vi "Readtext.vi"(8 "error in (no error)":errorcluster, 11 "object in":refnum<class "stream Message.lvclass">) -> (0 "error out":errorcluster, 2 "text":string, 3 "object out":refnum<class "stream Message.lvclass">)   [LabVIEW 2018, in "ClientMessaging.lvlib" / "stream Message.lvclass"]
uses:
  stream Message.lvclass
  stream Message.lvclass/stream Message.ctl
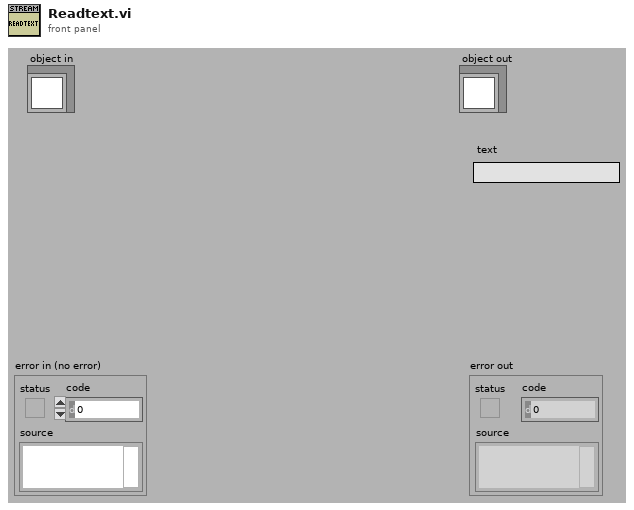
[diagram p1: front panel]
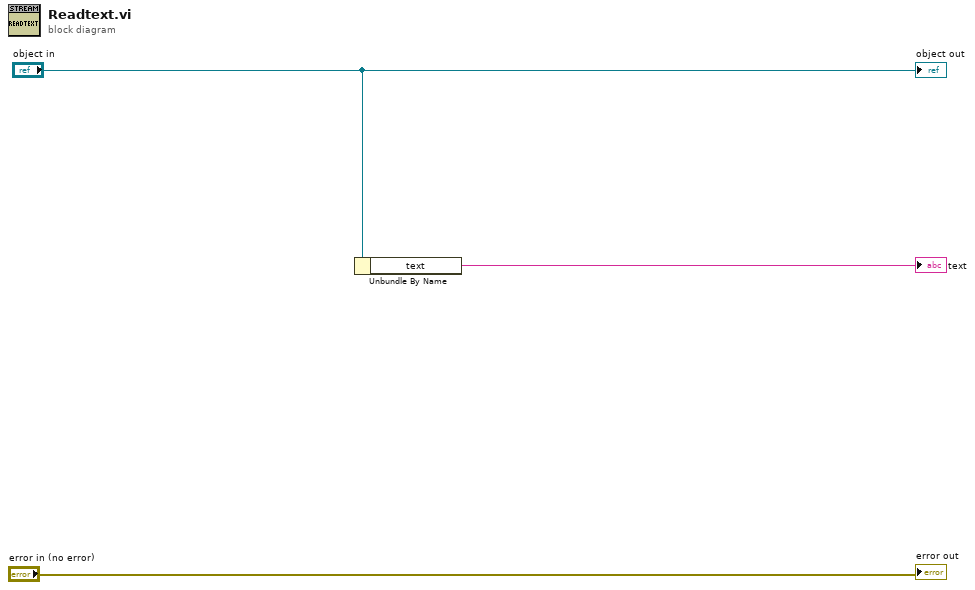
[diagram p0: block diagram]
diagram:
  n1 = Unbundle By Name("object in") -> ("text"=→"text":string)
  "error out" <- "error in (no error)"
  "object out" <- "object in"
